vi "抓邊_線.vi"(0 "Image In":T1, 1 "Process":T7(ring), 2 "Optimized Mode":bool, 3 "Direction":enum16{"Start to End", "End to Start"}(ring), 5 "ROI":T3, 11 "error In":errorcluster, 12 "Edge Options":T5={"Edge Polarity"=0, "Kernel Size"=3, "Width"=3, "Minimum Edge Strength"=10.0, "Interpolation Type"=enum."Bilinear Fixed", "Data Processing Method"=enum."Average"} {"Edge Polarity" items=["All Edges", "Rising Edges", "Falling Edges"]; "Minimum Edge Strength" format="%.2f"; "Width" step=2; "Kernel Size" step=2}, 13 "Point Diameter (5)":u32=5 min=3 max=1000) -> (4 "Image Out":T1, 6 "Line Profile":T4(graph), 10 "Gradient Information":dbl[][](graph), 14 "Location (Pixel)":cluster{"X":sgl, "Y":sgl}, 15 "error out":errorcluster)   [LabVIEW 2015]
uses:
  <vilib>/vision/Measure.llb/Edge Options.ctl
  <vilib>/vision/Measure.llb/Edge Polarity.ctl
  <vilib>/vision/Image Controls.llb/IMAQ Image.ctl
  <vilib>/vision/NI_Vision_Development_Module.lvlib
panel:
  out "Line":T2 {"Start X" scale=0.0..1024.0; "End X" scale=0.0..1024.0}
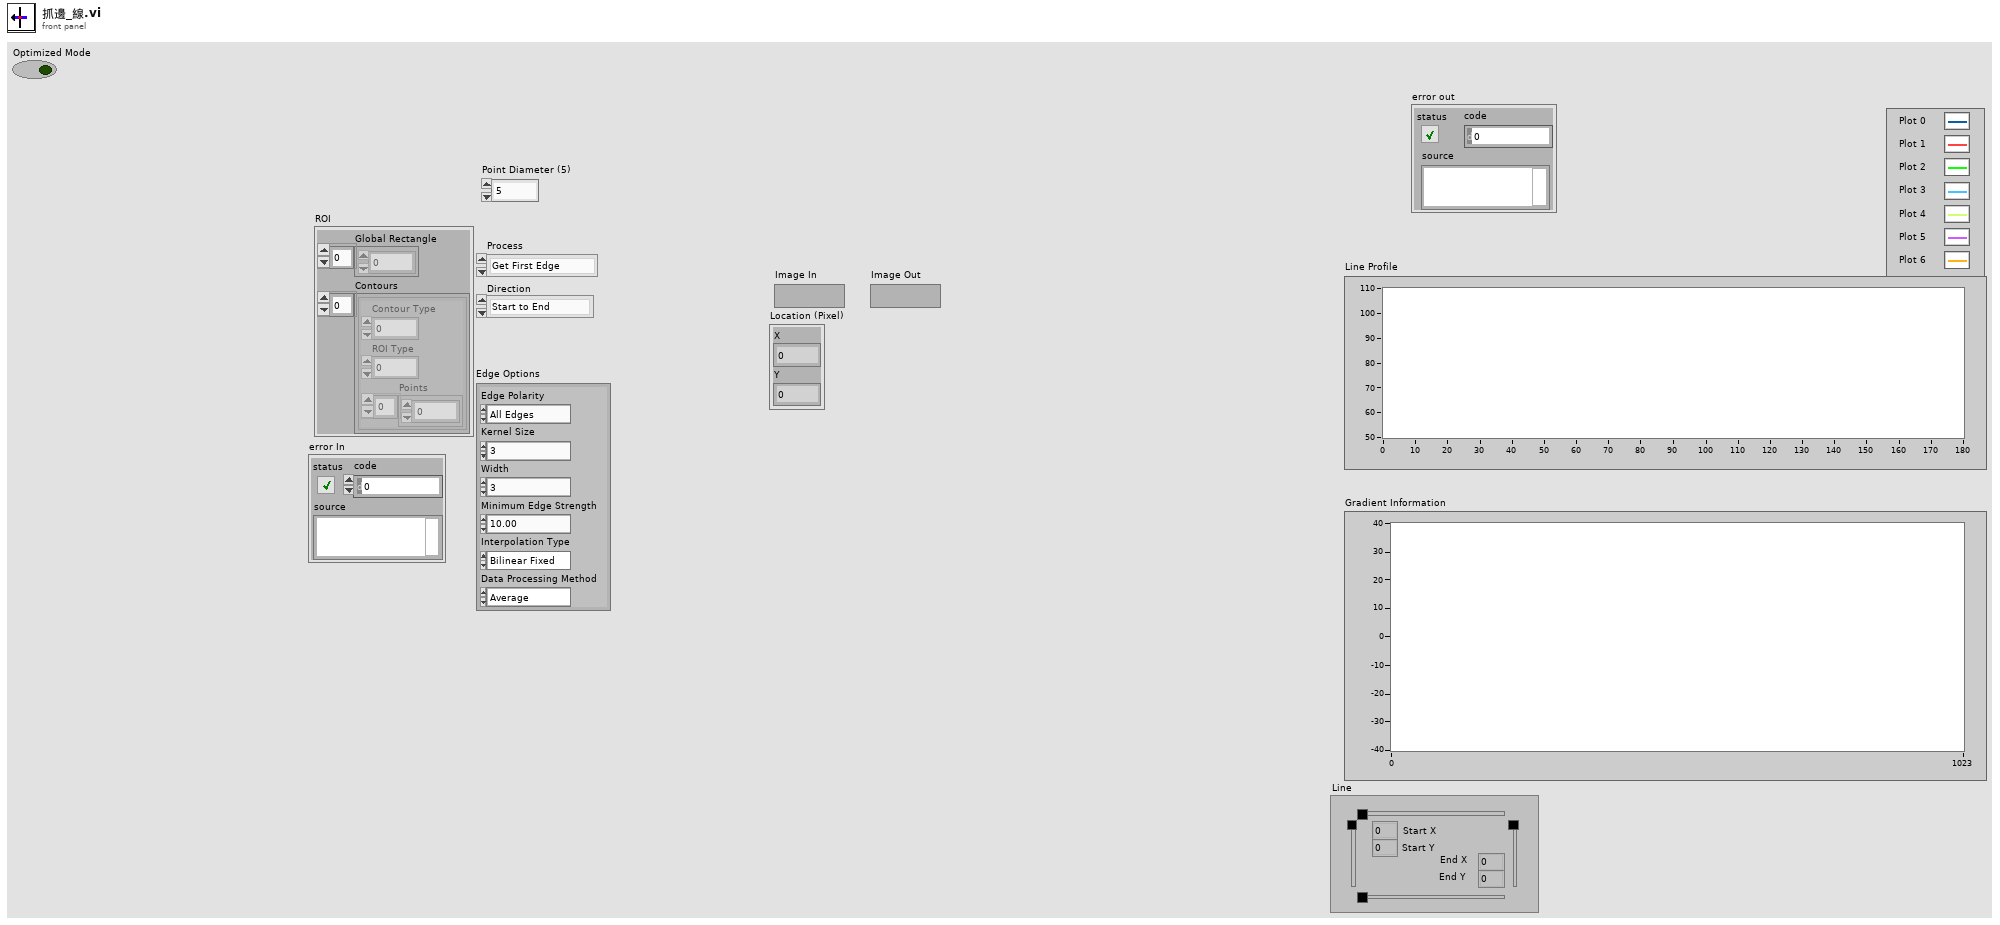
[diagram p1: front panel]
types:
  T1 = typedef "IMAQ Image.ctl" = refnum<image>
  T2 = typedef "IMAQ Line" = cluster{"Start X":i32, "Start Y":i32, "End X":i32, "End Y":i32}
  T3 = cluster{"Global Rectangle":i32[], "Contours":cluster{"Contour Type":u32, "ROI Type":u32, "Points":i32[]}[]}
  T4 = cluster{"x0":sgl, "dx":sgl, "Pixels Line":sgl[]}[]
  T5 = typedef "Edge Options.ctl" = cluster{"Edge Polarity":T6, "Kernel Size":u32, "Width":u32, "Minimum Edge Strength":sgl, "Interpolation Type":enum32{"Zero Order", "Bilinear", "Quadratic", "Cubic", "Bilinear Fixed"}, "Data Processing Method":enum32{"Average", "Median"}}
  T6 = typedef "Edge Polarity.ctl" = u32
  T7 = enum16{"Get First Edge", "Get First + Last Edge", "Get All Edges", "Get Best Edge"}
  T8 = cluster{"Point 1":cluster{"x":dbl, "y":dbl}, "Point 2":cluster{"x":dbl, "y":dbl}}
  T9 = typedef "ROI Descriptor" = cluster{"Global Rectangle":i32[], "Contours":cluster{"ID":enum32{"External", "Internal"}, "Type":u32, "Coordinates":i32[]}[]}
  T10 = typedef "Edge New.ctl" = cluster{"Location (Pixel)":cluster{"X":sgl, "Y":sgl}, "Location (Real-World)":cluster{"X":sgl, "Y":sgl}, "Distance (Pixel)":dbl, "Distance (Real-World)":dbl, "Strength":dbl, "Noise":dbl, "Rising?":bool}
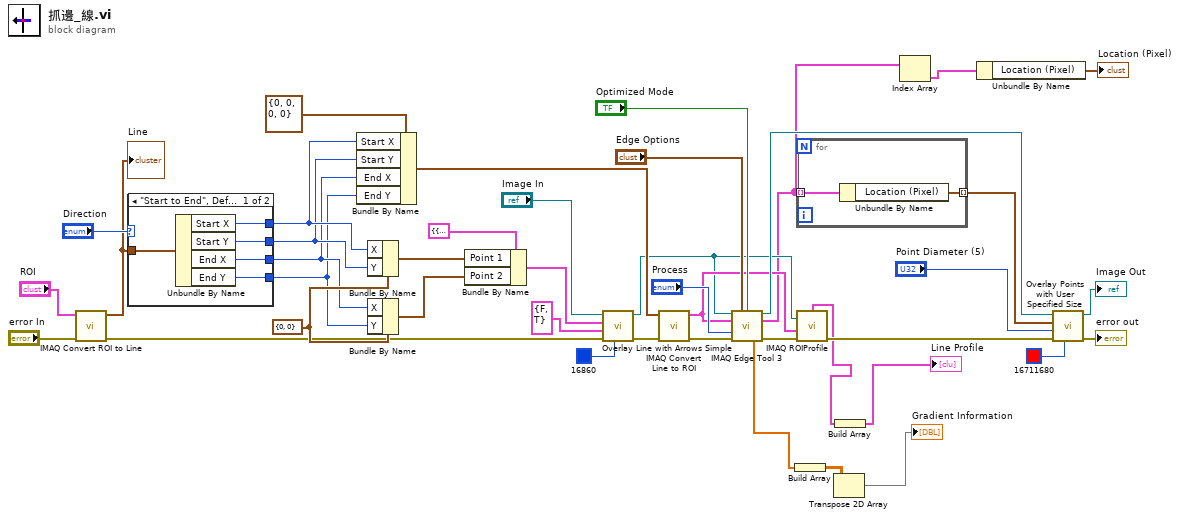
[diagram p0: block diagram]
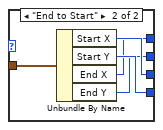
[diagram p2: hidden frame]
diagram:
  w19 = cluster{"X":i32, "Y":i32} {"X"=0, "Y"=0} ("Start Point")
  n1 = call "IMAQ Convert ROI to Line"("error in (no error)"="error In", "ROI Descriptor"="ROI") -> ("error out"=w9:errorcluster, "Line"=w39:T2)  [unwired: 7 in]
  "Line" <- w39
  n2 = case shown="\"Start to End\", Default" "Direction" {
    tunnel: w39 -> [w47 w48]
    tunnel: [w46 w50] -> w17
    tunnel: [w45 w49] -> w16
    tunnel: [w44 w52] -> w15
    tunnel: [w43 w51] -> w14
    frame "Start to End", Default {
      n3 = Unbundle By Name(w47) -> ("Start X"=w46:i32, "Start Y"=w45:i32, "End X"=w44:i32, "End Y"=w43:i32)
    }
    frame "End to Start" {
      n4 = Unbundle By Name(w48) -> ("Start X"=w52:i32, "Start Y"=w51:i32, "End X"=w50:i32, "End Y"=w49:i32)
    }
  }
  n5 = Bundle By Name(cluster=T2 {"Start X"=0, "Start Y"=0, "End X"=0, "End Y"=0} ("Line"), "Start X"=w17, "Start Y"=w16, "End X"=w15, "End Y"=w14) -> (w29:T2)
  n6 = Bundle By Name(cluster=w19, "X"=w17, "Y"=w16) -> (w20:cluster{"X":i32, "Y":i32})
  n7 = Bundle By Name(cluster=w19, "X"=w15, "Y"=w14) -> (w18:cluster{"X":i32, "Y":i32})
  n8 = Bundle By Name(cluster=T8 {"Point 1"={"x"=50.0, "y"=50.0}, "Point 2"={"x"=70.0, "y"=70.0}} ("Line Coordinates"), "Point 1"=w20, "Point 2"=w18) -> (w26:T8)
  n9 = call "Overlay Line with Arrows Simple.vi"("Color"=u32 16860, "error in"=w9, "Arrows"=cluster{"Start point":bool, "End point":bool} {"Start point"=FALSE, "End point"=TRUE}, "Line Coordinates"=w26, "Image In"="Image In") -> ("error out"=w24:errorcluster, "Image Out"=w25:T1)  [unwired: 5 in]
  n10 = call "IMAQ Convert Line to ROI"("error in (no error)"=w24, "Line"=w29) -> ("error out"=w33:errorcluster, "ROI Descriptor"=w32:T9)  [unwired: 7 in]
  n11 = call "IMAQ Edge Tool 3"("Image"=w25, "Edge Options"="Edge Options", "Optimized Mode"="Optimized Mode", "ROI Descriptor"=w32, "Process"="Process", "error in (no error)"=w33) -> ("Image (duplicate)"=w35:T1, "Edge Information"=w5:T10[], "Gradient Values"=w8:dbl[], "error out"=w34:errorcluster)  [unwired: 5 in, 1 out]
  n12 = Build Array(w8) -> (w7:dbl[][])
  n13 = for {
    tunnel: w5 -> [w54] mode=indexing
    tunnel: [w53] -> w22 mode=indexing
    n14 = Unbundle By Name(w54) -> ("Location (Pixel)"=w53:cluster{"X":sgl, "Y":sgl})
  }
  n15 = call "IMAQ ROIProfile"("error in (no error)"=w34, "ROI Descriptor"=w32, "Image"=w25) -> ("error out"=w37:errorcluster, "ROI Graph"=w2:cluster{"x0":sgl, "dx":sgl, "Pixels Line":sgl[]})  [unwired: 1 in, 3 out]
  n16 = Transpose 2D Array(2D array=w7) -> (transposed array=→"Gradient Information":dbl[][])
  n17 = Build Array(w2) -> (→"Line Profile":T4)
  n18 = Index Array(array=w5) -> (element=w4:T10)  [unwired: 1 in]
  n19 = Unbundle By Name(w4) -> ("Location (Pixel)"=→"Location (Pixel)":cluster{"X":sgl, "Y":sgl})
  n20 = call "Overlay Points with User Specified Size.vi"("Color"=u32 16711680, "error in"=w37, "Point Diameter (5)"="Point Diameter (5)", "Points"=w22, "Image In"=w35) -> ("error out"=→"error out":errorcluster, "Image Out"=→"Image Out":T1)  [unwired: 5 in]
